vi "Edit-action-in-sequence.vi"(5 "Sequence index in":i32, 7 "Motor index":i32, 8 "error in (no error)":errorcluster, 11 "Available motors in":refnum<class "Motor-assembly.lvclass">) -> (0 "error out":errorcluster, 3 "Available motors out":refnum<class "Motor-assembly.lvclass">, 4 "Sequence index":i32)   [LabVIEW 2013, in "PowderDeposition.lvlib" / "Motor-assembly.lvclass"]
uses:
  Motor-assembly.lvclass
  Motor-assembly.lvclass/Motor-assembly.ctl
  Motor/Motor.lvclass
  Sequence/Action-sequence.lvclass
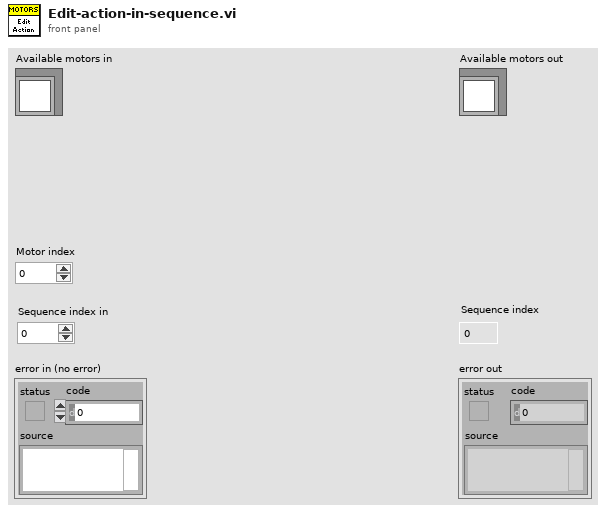
[diagram p1: front panel]
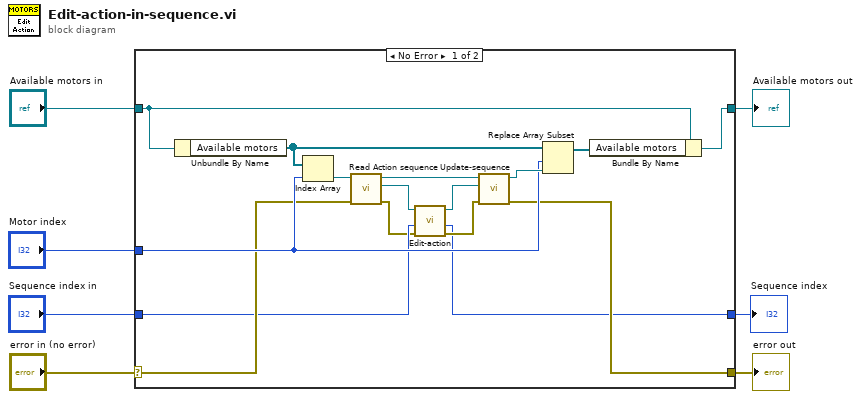
[diagram p0: block diagram]
diagram:
  n1 = case shown="No Error" "error in (no error)" {
    selector: "error in (no error)" -> [w15 w26]
    tunnel: [w14 w26] -> w6
    tunnel: [w18 w25] -> w4
    tunnel: "Available motors in" -> [w19 w25]
    tunnel: "Motor index" -> [w17 _]
    tunnel: "Sequence index in" -> [w9 w24]
    tunnel: [w10 w24] -> w1
    frame No Error {
      n2 = Unbundle By Name(w19) -> ("Available motors"=w16:refnum<class "Motor.lvclass">[])
      n3 = Index Array(array=w16, index=w17) -> (element=w21:refnum<class "Motor.lvclass">)
      n4 = call-dynamic "Read Action sequence.vi"("error in (no error)"=w15, "Motor in"=w21) -> ("error out"=w8:errorcluster, "Sequence.lvclass"=w13:refnum<class "Action-sequence.lvclass">, "Motor out"=w22:refnum<class "Motor.lvclass">)  [unwired: 7 in]
      n5 = call "Edit-action.vi"("error in (no error)"=w8, "Position in"=w9, "Sequence in"=w13) -> ("error out"=w11:errorcluster, "Position"=w10:i32, "Sequence out"=w12:refnum<class "Action-sequence.lvclass">)  [unwired: 6 in]
      n6 = call-dynamic "Update-sequence.vi"("error in (no error)"=w11, "Sequence"=w12, "Motor in"=w22) -> ("error out"=w14:errorcluster, "Motor out"=w23:refnum<class "Motor.lvclass">)  [unwired: 7 in]
      n7 = Replace Array Subset(array=w16, new element=w23, index=w17) -> (w20:refnum<class "Motor.lvclass">[])
      n8 = Bundle By Name(cluster=w19, "Available motors"=w20) -> (w18:refnum<class "Motor-assembly.lvclass">)
    }
    frame Error {
    }
  }
  "error out" <- w6
  "Available motors out" <- w4
  "Sequence index" <- w1
